vi "ReadData9234.vi"(8 "error in":errorcluster, 11 "Module Config Selector":i16) -> (0 "error out":errorcluster, 3 "Data Array":sgl[](array[numeric]) format="%.2f")   [LabVIEW 2017, in "BOP_VibAPI_6.lvlib"]
uses:
  <vilib>/addons/InsightCM/Devices/Shared/Cms/Fpga/Acquisition/source/subVIs/VibAPI/BOP_VibAPI_6.lvlib
  <vilib>/rvi/eio/common/nirviEmuTemplateMethod_errors.vi
  <vilib>/eio/EIONode/EIONode.xnode
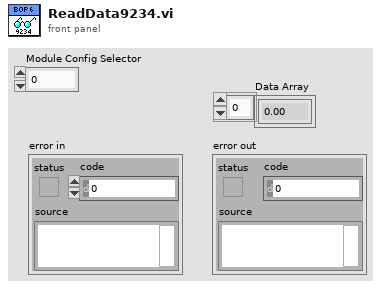
[diagram p1: front panel]
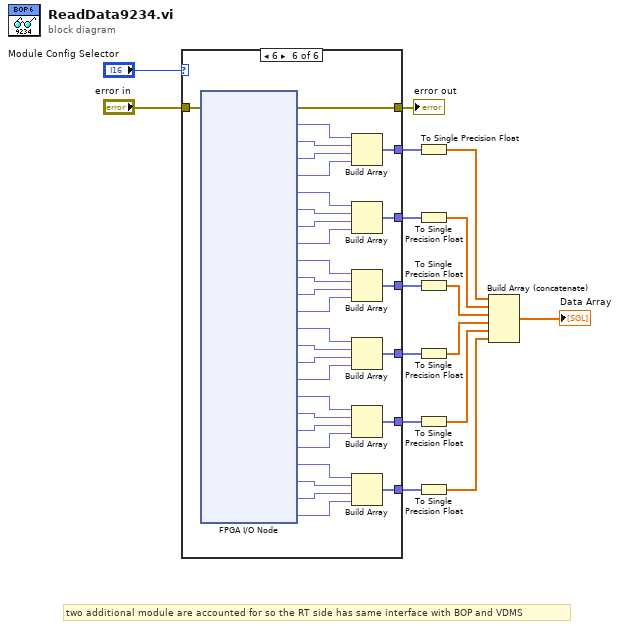
[diagram p0: block diagram]
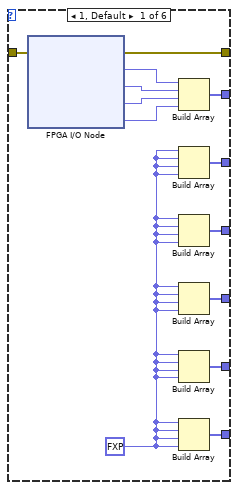
[diagram p2: hidden frame]
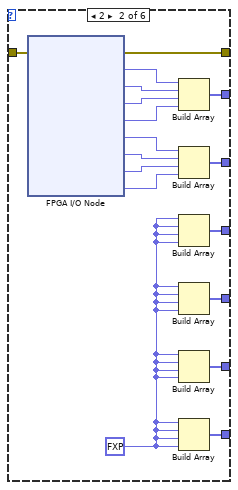
[diagram p3: hidden frame]
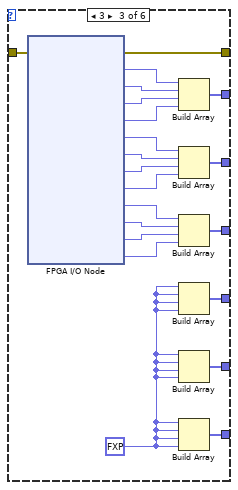
[diagram p4: hidden frame]
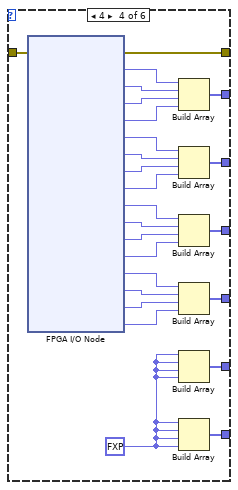
[diagram p5: hidden frame]
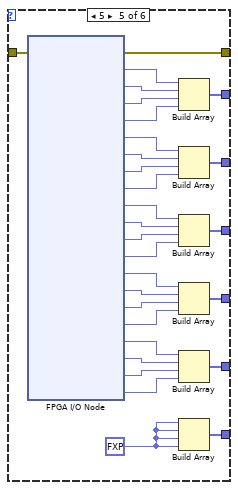
[diagram p6: hidden frame]
diagram:
  # "two additional module are accounted for so the RT side has same interface with BOP and VDMS"
  n1 = case shown="6" "Module Config Selector" {
    tunnel: "error in" -> [w26 w43 w64 w89 w118 w150]
    tunnel: [w25 w42 w63 w88 w117 w149] -> w15
    tunnel: [w24 w41 w62 w87 w116 w148] -> w13
    tunnel: [w23 w40 w61 w86 w115 w147] -> w10
    tunnel: [w22 w39 w60 w85 w114 w146] -> w9
    tunnel: [w18 w31 w48 w84 w113 w145] -> w8
    tunnel: [w21 w38 w59 w83 w112 w144] -> w7
    tunnel: [w20 w37 w58 w82 w111 w143] -> w6
    frame 1, Default {
      w17 = fxp<+/-,24,7> 0.0 ("Mod1/AI2")
      n2 = xnode "FPGA I/O Node"("error in"=w26) -> ("error out"=w25:errorcluster, "Mod1/AI0"=w27:fxp<+/-,24,4>, "Mod1/AI1"=w29:fxp<+/-,24,4>, "Mod1/AI2"=w28:fxp<+/-,24,4>, "Mod1/AI3"=w19:fxp<+/-,24,4>)  [unwired: 4 in, 4 out]
      n3 = Build Array(w27, w29, w28, w19) -> (w24:fxp<+/-,24,4>[])
      n4 = Build Array(w17, w17, w17, w17) -> (w23:fxp<+/-,24,7>[])
      n5 = Build Array(w17, w17, w17, w17) -> (w22:fxp<+/-,24,7>[])
      n6 = Build Array(w17, w17, w17, w17) -> (w18:fxp<+/-,24,7>[])
      n7 = Build Array(w17, w17, w17, w17) -> (w21:fxp<+/-,24,7>[])
      n8 = Build Array(w17, w17, w17, w17) -> (w20:fxp<+/-,24,7>[])
    }
    frame 2 {
      w30 = fxp<+/-,24,7> 0.0 ("Mod1/AI2")
      n9 = xnode "FPGA I/O Node"("error in"=w43) -> ("error out"=w42:errorcluster, "Mod1/AI0"=w44:fxp<+/-,24,4>, "Mod1/AI1"=w46:fxp<+/-,24,4>, "Mod1/AI2"=w45:fxp<+/-,24,4>, "Mod1/AI3"=w33:fxp<+/-,24,4>, "Mod2/AI0"=w36:fxp<+/-,24,4>, "Mod2/AI1"=w35:fxp<+/-,24,4>, "Mod2/AI2"=w34:fxp<+/-,24,4>, "Mod2/AI3"=w32:fxp<+/-,24,4>)  [unwired: 8 in, 8 out]
      n10 = Build Array(w44, w46, w45, w33) -> (w41:fxp<+/-,24,4>[])
      n11 = Build Array(w36, w35, w34, w32) -> (w40:fxp<+/-,24,4>[])
      n12 = Build Array(w30, w30, w30, w30) -> (w39:fxp<+/-,24,7>[])
      n13 = Build Array(w30, w30, w30, w30) -> (w31:fxp<+/-,24,7>[])
      n14 = Build Array(w30, w30, w30, w30) -> (w38:fxp<+/-,24,7>[])
      n15 = Build Array(w30, w30, w30, w30) -> (w37:fxp<+/-,24,7>[])
    }
    frame 3 {
      w47 = fxp<+/-,24,7> 0.0 ("Mod1/AI2")
      n16 = xnode "FPGA I/O Node"("error in"=w64) -> ("error out"=w63:errorcluster, "Mod1/AI0"=w65:fxp<+/-,24,4>, "Mod1/AI1"=w67:fxp<+/-,24,4>, "Mod1/AI2"=w66:fxp<+/-,24,4>, "Mod1/AI3"=w51:fxp<+/-,24,4>, "Mod2/AI0"=w57:fxp<+/-,24,4>, "Mod2/AI1"=w56:fxp<+/-,24,4>, "Mod2/AI2"=w55:fxp<+/-,24,4>, "Mod2/AI3"=w49:fxp<+/-,24,4>, "Mod3/AI0"=w54:fxp<+/-,24,4>, "Mod3/AI1"=w53:fxp<+/-,24,4>, "Mod3/AI2"=w52:fxp<+/-,24,4>, "Mod3/AI3"=w50:fxp<+/-,24,4>)  [unwired: 12 in, 12 out]
      n17 = Build Array(w65, w67, w66, w51) -> (w62:fxp<+/-,24,4>[])
      n18 = Build Array(w57, w56, w55, w49) -> (w61:fxp<+/-,24,4>[])
      n19 = Build Array(w54, w53, w52, w50) -> (w60:fxp<+/-,24,4>[])
      n20 = Build Array(w47, w47, w47, w47) -> (w48:fxp<+/-,24,7>[])
      n21 = Build Array(w47, w47, w47, w47) -> (w59:fxp<+/-,24,7>[])
      n22 = Build Array(w47, w47, w47, w47) -> (w58:fxp<+/-,24,7>[])
    }
    frame 4 {
      w68 = fxp<+/-,24,7> 0.0 ("Mod1/AI2")
      n23 = xnode "FPGA I/O Node"("error in"=w89) -> ("error out"=w88:errorcluster, "Mod1/AI0"=w90:fxp<+/-,24,4>, "Mod1/AI1"=w92:fxp<+/-,24,4>, "Mod1/AI2"=w91:fxp<+/-,24,4>, "Mod1/AI3"=w72:fxp<+/-,24,4>, "Mod2/AI0"=w81:fxp<+/-,24,4>, "Mod2/AI1"=w80:fxp<+/-,24,4>, "Mod2/AI2"=w79:fxp<+/-,24,4>, "Mod2/AI3"=w69:fxp<+/-,24,4>, "Mod3/AI0"=w78:fxp<+/-,24,4>, "Mod3/AI1"=w77:fxp<+/-,24,4>, "Mod3/AI2"=w76:fxp<+/-,24,4>, "Mod3/AI3"=w70:fxp<+/-,24,4>, "Mod4/AI0"=w75:fxp<+/-,24,4>, "Mod4/AI1"=w74:fxp<+/-,24,4>, "Mod4/AI2"=w73:fxp<+/-,24,4>, "Mod4/AI3"=w71:fxp<+/-,24,4>)  [unwired: 16 in, 16 out]
      n24 = Build Array(w90, w92, w91, w72) -> (w87:fxp<+/-,24,4>[])
      n25 = Build Array(w81, w80, w79, w69) -> (w86:fxp<+/-,24,4>[])
      n26 = Build Array(w78, w77, w76, w70) -> (w85:fxp<+/-,24,4>[])
      n27 = Build Array(w75, w74, w73, w71) -> (w84:fxp<+/-,24,4>[])
      n28 = Build Array(w68, w68, w68, w68) -> (w83:fxp<+/-,24,7>[])
      n29 = Build Array(w68, w68, w68, w68) -> (w82:fxp<+/-,24,7>[])
    }
    frame 5 {
      w93 = fxp<+/-,24,7> 0.0 ("Mod1/AI2")
      n30 = xnode "FPGA I/O Node"("error in"=w118) -> ("error out"=w117:errorcluster, "Mod1/AI0"=w119:fxp<+/-,24,4>, "Mod1/AI1"=w121:fxp<+/-,24,4>, "Mod1/AI2"=w120:fxp<+/-,24,4>, "Mod1/AI3"=w98:fxp<+/-,24,4>, "Mod2/AI0"=w110:fxp<+/-,24,4>, "Mod2/AI1"=w109:fxp<+/-,24,4>, "Mod2/AI2"=w108:fxp<+/-,24,4>, "Mod2/AI3"=w94:fxp<+/-,24,4>, "Mod3/AI0"=w107:fxp<+/-,24,4>, "Mod3/AI1"=w106:fxp<+/-,24,4>, "Mod3/AI2"=w105:fxp<+/-,24,4>, "Mod3/AI3"=w95:fxp<+/-,24,4>, "Mod4/AI0"=w104:fxp<+/-,24,4>, "Mod4/AI1"=w103:fxp<+/-,24,4>, "Mod4/AI2"=w102:fxp<+/-,24,4>, "Mod4/AI3"=w96:fxp<+/-,24,4>, "Mod5/AI0"=w101:fxp<+/-,24,4>, "Mod5/AI1"=w100:fxp<+/-,24,4>, "Mod5/AI2"=w99:fxp<+/-,24,4>, "Mod5/AI3"=w97:fxp<+/-,24,4>)  [unwired: 20 in, 20 out]
      n31 = Build Array(w119, w121, w120, w98) -> (w116:fxp<+/-,24,4>[])
      n32 = Build Array(w110, w109, w108, w94) -> (w115:fxp<+/-,24,4>[])
      n33 = Build Array(w107, w106, w105, w95) -> (w114:fxp<+/-,24,4>[])
      n34 = Build Array(w104, w103, w102, w96) -> (w113:fxp<+/-,24,4>[])
      n35 = Build Array(w101, w100, w99, w97) -> (w112:fxp<+/-,24,4>[])
      n36 = Build Array(w93, w93, w93, w93) -> (w111:fxp<+/-,24,7>[])
    }
    frame 6 {
      n37 = xnode "FPGA I/O Node"("error in"=w150) -> ("error out"=w149:errorcluster, "Mod1/AI0"=w151:fxp<+/-,24,4>, "Mod1/AI1"=w153:fxp<+/-,24,4>, "Mod1/AI2"=w152:fxp<+/-,24,4>, "Mod1/AI3"=w127:fxp<+/-,24,4>, "Mod2/AI0"=w142:fxp<+/-,24,4>, "Mod2/AI1"=w141:fxp<+/-,24,4>, "Mod2/AI2"=w140:fxp<+/-,24,4>, "Mod2/AI3"=w122:fxp<+/-,24,4>, "Mod3/AI0"=w139:fxp<+/-,24,4>, "Mod3/AI1"=w138:fxp<+/-,24,4>, "Mod3/AI2"=w137:fxp<+/-,24,4>, "Mod3/AI3"=w123:fxp<+/-,24,4>, "Mod4/AI0"=w136:fxp<+/-,24,4>, "Mod4/AI1"=w135:fxp<+/-,24,4>, "Mod4/AI2"=w134:fxp<+/-,24,4>, "Mod4/AI3"=w124:fxp<+/-,24,4>, "Mod5/AI0"=w133:fxp<+/-,24,4>, "Mod5/AI1"=w132:fxp<+/-,24,4>, "Mod5/AI2"=w131:fxp<+/-,24,4>, "Mod5/AI3"=w125:fxp<+/-,24,4>, "Mod6/AI0"=w130:fxp<+/-,24,4>, "Mod6/AI1"=w129:fxp<+/-,24,4>, "Mod6/AI2"=w128:fxp<+/-,24,4>, "Mod6/AI3"=w126:fxp<+/-,24,4>)  [unwired: 24 in, 24 out]
      n38 = Build Array(w151, w153, w152, w127) -> (w148:fxp<+/-,24,4>[])
      n39 = Build Array(w142, w141, w140, w122) -> (w147:fxp<+/-,24,4>[])
      n40 = Build Array(w139, w138, w137, w123) -> (w146:fxp<+/-,24,4>[])
      n41 = Build Array(w136, w135, w134, w124) -> (w145:fxp<+/-,24,4>[])
      n42 = Build Array(w133, w132, w131, w125) -> (w144:fxp<+/-,24,4>[])
      n43 = Build Array(w130, w129, w128, w126) -> (w143:fxp<+/-,24,4>[])
    }
  }
  "error out" <- w15
  n44 = To Single Precision Float(number=w13) -> (single precision float=w12:sgl[])
  n45 = To Single Precision Float(number=w10) -> (single precision float=w5:sgl[])
  n46 = To Single Precision Float(number=w9) -> (single precision float=w4:sgl[])
  n47 = To Single Precision Float(number=w8) -> (single precision float=w3:sgl[])
  n48 = To Single Precision Float(number=w7) -> (single precision float=w2:sgl[])
  n49 = To Single Precision Float(number=w6) -> (single precision float=w1:sgl[])
  n50 = Build Array (concatenate)(w12, w5, w4, w3, w2, w1) -> (→"Data Array":sgl[])
